vi "Set Power Supplies On.vi"(8 "error in (no error)":errorcluster, 9 "Power On":bool, 10 "Active Positions":u32, 11 "Driver Test":refnum<class "Driver Test.lvclass">) -> (0 "error out":errorcluster)   [LabVIEW 2015, in "Driver Test.lvclass"]
doc: "Switches <b>Position</b> to <b>Power On</b>, than sets the power supply and dimming to base values from the recipe."
uses:
  Driver Test.lvclass
  Test Class/Test Class.lvclass
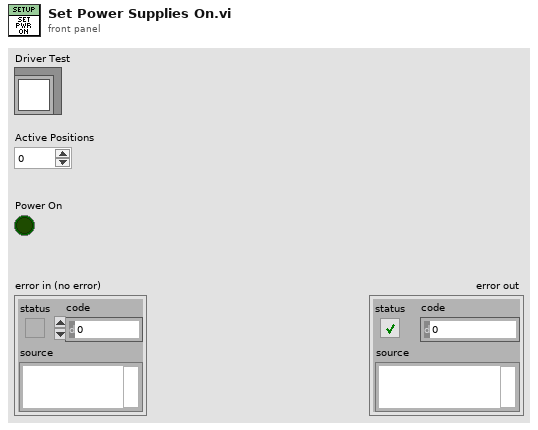
[diagram p1: front panel]
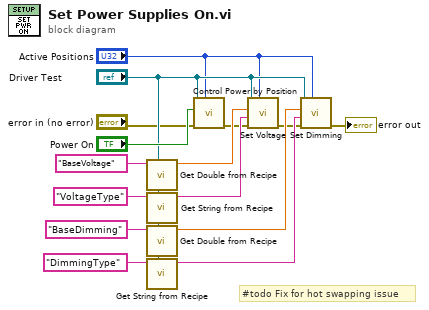
[diagram p0: block diagram]
diagram:
  # "#todo Fix for hot swapping issue"
  n1 = call "Get Double from Recipe.vi"("Test Class in"="Driver Test", "Name"="BaseVoltage") -> ("Value"=w14:dbl)  [unwired: 7 in, 2 out]
  n2 = call "Get String from Recipe.vi"("Test Class in"="Driver Test", "Name"="VoltageType") -> ("Value"=w11:string)  [unwired: 7 in, 2 out]
  n3 = call "Get Double from Recipe.vi"("Test Class in"="Driver Test", "Name"="BaseDimming") -> ("Value"=w12:dbl)  [unwired: 7 in, 2 out]
  n4 = call "Get String from Recipe.vi"("Test Class in"="Driver Test", "Name"="DimmingType") -> ("Value"=w13:string)  [unwired: 7 in, 2 out]
  n5 = call "Control Power by Position.vi"("Position"="Active Positions", "error in (no error)"="error in (no error)", "Power On?"="Power On", "Driver Test in"="Driver Test") -> ("error out"=w3:errorcluster)  [unwired: 7 in]
  n6 = call "Set Voltage.vi"("Position"="Active Positions", "error in (no error)"=w3, "Voltage Type"=w11, "Voltage"=w14, "Driver Test in"="Driver Test") -> ("error out"=w4:errorcluster)  [unwired: 6 in]
  n7 = call "Set Dimming.vi"("Position"="Active Positions", "error in (no error)"=w4, "Dimming Type"=w13, "Dim Level"=w12, "Driver Test in"="Driver Test") -> ("error out"=→"error out":errorcluster)  [unwired: 6 in]
